vi "Vision Processing.vi"(8 "error in (no error)":errorcluster, 11 "Image Size":T2=enum."320x240") -> ()   [LabVIEW 2019]
uses:
  Vision Support Code/Camera Types.ctl
  <vilib>/Rock Robotics/WPI/Camera/WPI_CameraImageSize.ctl
  <vilib>/Rock Robotics/WPI/Camera/WPI_CameraWhite Balance Values.ctl
  <vilib>/Rock Robotics/WPI/Camera/WPI_CameraExposure Values.ctl
  <vilib>/Rock Robotics/WPI/Camera/WPI_CameraFrameRate.ctl
  Robot Global Data.vi
  <vilib>/Rock Robotics/Network Tables/NT Write Variant.vi
  <vilib>/vision/NI_Vision_Development_Module.lvlib
panel:
  out "Disqualified":i32
  out "Results":T1(array[cluster]) {"Normalized Center"."x" format="%#_2g"; "Normalized Center"."y" format="%#_2g"; "Overall Score" format="%#_2g"; "Distance (ft)" format="%#_3g"; "Area Score" format="%#_2g"; "Moment Score" format="%#_2g"; "Aspect Score" format="%#_2g"}
  in  "Size Limit %":dbl=0.04
  out "loop ms":u32
  in  "Display Original":bool
  in  "Display Mask":bool
  out "Instructions:":string="Connect a USB or IP camera to your roboRIO. If using a ring light and retroreflective tape, use Camera Settings outside the loop create a dark image with bright and colorful stripes. If used wihtout a ring light, brighten the images so that stripes are visible.\n\nLED Color can encoded as HSL or related color modes. Calibrate to the same color as the strips being reflected to the camera. Unlike the desktop example, this LED color must be set by hand. You can also put the calibration on the dashboard and send the LED Color to the RT code using Network Tables.\n\nThe Display buttons affects whether images are displayed on the panel. It takes quite a bit of CPU  to compress and transmit the images for display.\n\nAdjust Score Cutoff to make the code more or less picky. If the color is not very unique, you may need to increase the number of particles considered. The diagram uses a Size Limit to ignore colored things that are too small. You may need to adjust it if you are targetting from far away.\n\nResults give you the distance to the target, the center and box in a normalized (-1 to 1) and pixel coordinates.\n\nBe sure to read about setting camera exposure and brightness to help simplify your image and acquire color saturated images.\n\nThere are lots of comments on the diagram to explain the code."
  in  "Color Mode":u16(ring)=2 items=["RGB", "HSL", "HSV", "HSI"]
  in  "Particles":dbl=5.0
  in  "Score Cutoff %":dbl=75.0
  in  "Camera Type":T3=enum."MS HD3000 square"
  out "Qualified":i32
  in  "LED Color":T4={"Hue"={107.81818389892578, 139.81818389892578}, "Sat"={176.07142857142858, 255.0}, "Val"={40.53571428571429, 255.0}} {"Hue" scale=0.0..255.0 scale format="%#_3g"}
  out "Mask":T5(plugin-control)
  out "Original Image":T5(plugin-control)
  # "Scores"
  # "Good target, distance ft"
  # "Bad target"
  # "Score in %"
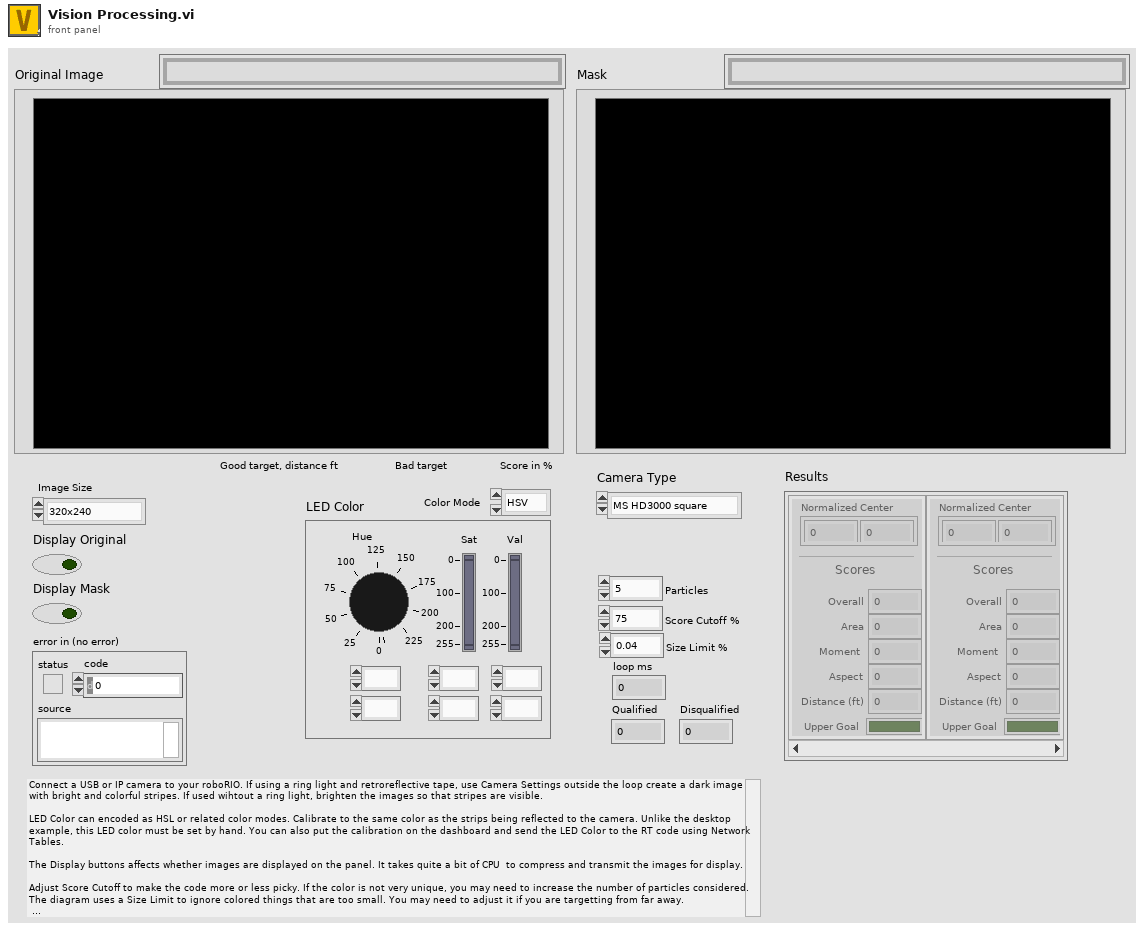
[diagram p1: front panel]
types:
  T1 = cluster{"diameter points":cluster{"first point":cluster{"x":dbl, "y":dbl}, "projected point":cluster{"x":dbl, "y":dbl}}, "Normalized Center":cluster{"x":dbl, "y":dbl}, "Overall Score":dbl, "Area Score":dbl, "Moment Score":dbl, "Aspect Score":dbl, "Distance (ft)":dbl, "Upper Goal":bool}[]
  T2 = typedef "WPI_CameraImageSize.ctl" = enum16{"640x480", "320x240", "160x120", "Custom"}
  T3 = typedef "Camera Types.ctl" = enum16{"206", "1011", "1013", "MS HD3000 square", "MS HD3000 640x480"}
  T4 = cluster{"Hue":cluster{dbl, dbl}, "Sat":cluster{dbl, dbl}, "Val":cluster{dbl, dbl}}
  T5 = typedef "IMAQ Image.ctl" = refnum<image>
  T6 = typedef "WPI_CameraFrameRate.ctl" = u32
  T7 = typedef "WPI_CameraExposure Values.ctl" = enum16{"Auto", "Flicker-free 50 Hz", "Flicker-free 60 Hz", "Hold current", "Custom"}
  T8 = typedef "WPI_CameraWhite Balance Values.ctl" = enum16{"Auto", "Fixed indoor", "Fixed outdoor 1", "Fixed outdoor 2", "Fixed fluorescent 1", "Fixed fluorescent 2", "Hold current", "Custom"}
  T9 = typedef "Particle Parameters" = i32
  T10 = typedef "Image Type" = u32
  T11 = typedef "WPI_CameraDevRef.ctl" = cluster{"Camera Address":string, "CameraStatus":errorcluster}
  T12 = cluster{"remainder":i32, "size":bool, "count":bool}
  T13 = typedef "Target Fields.ctl" = cluster{"diameter points":cluster{"first point":cluster{"x":dbl, "y":dbl}, "projected point":cluster{"x":dbl, "y":dbl}}, "normalized center":cluster{"x":dbl, "y":dbl}, "Overall Score":dbl, "Area Score":dbl, "Moment Score":dbl, "Aspect Score":dbl, "Distance (ft)":dbl, "Upper Goal":bool}
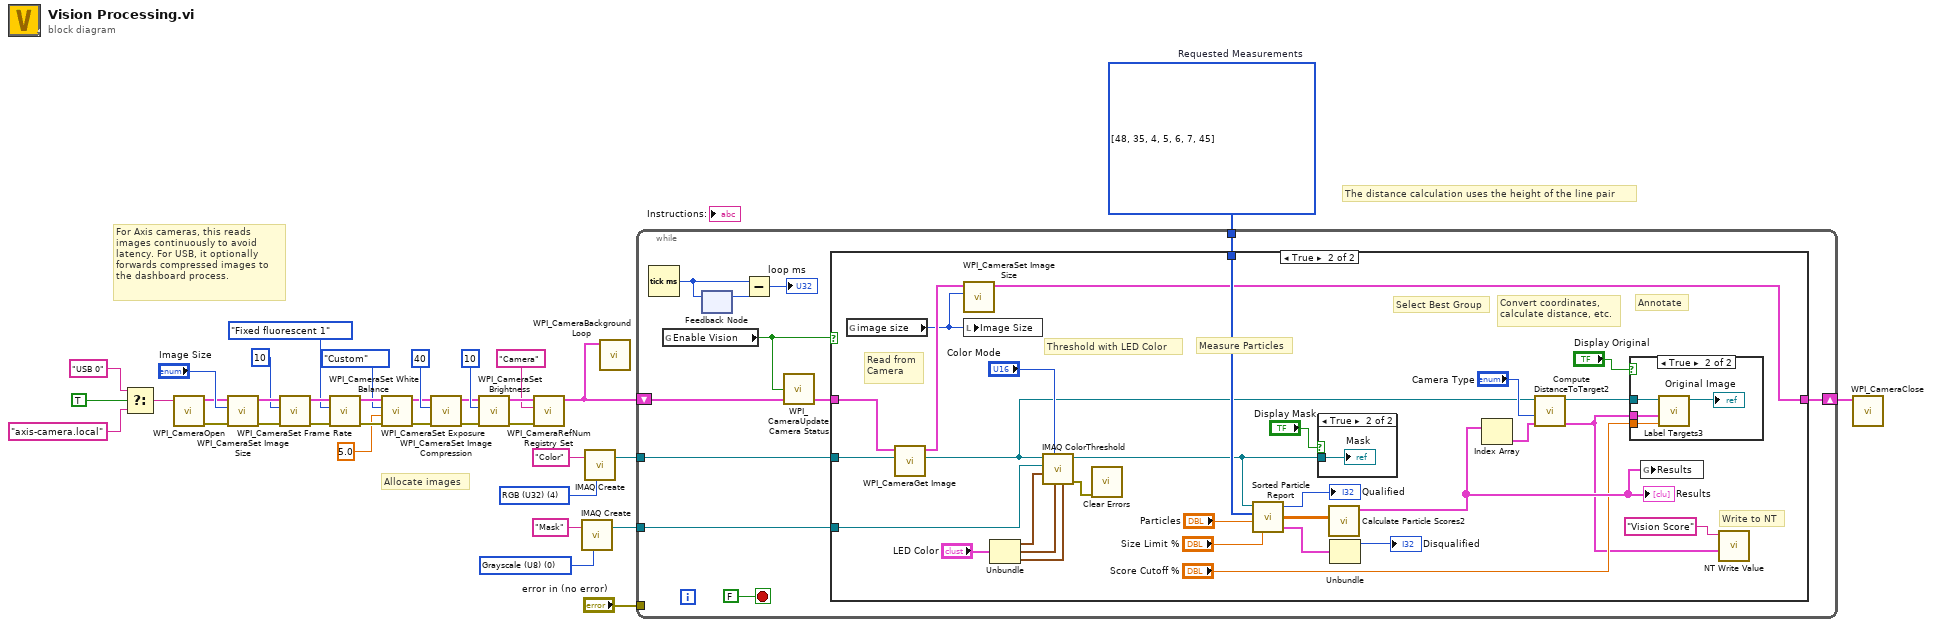
[diagram p0: block diagram]
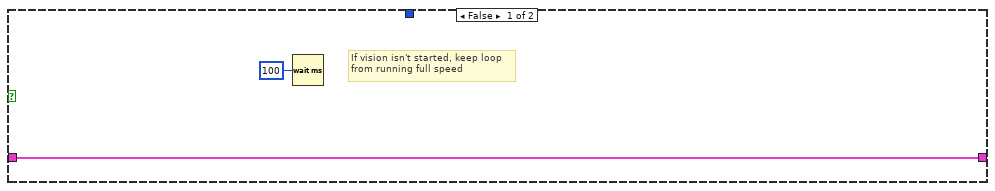
[diagram p2: hidden frame]
diagram:
  w31 = T9[] [48, 35, 4, 5, 6, 7, 45] items=["Center of Mass X", "Center of Mass Y", "First Pixel X", "First Pixel Y", "Bounding Rect Left", "Bounding Rect Top", "Bounding Rect Right", "Bounding Rect Bottom", "Max Feret Diameter Start X", "Max Feret Diameter Start Y", "Max Feret Diameter End X", "Max Feret Diameter End Y", "Max Horiz. Segment Length Left", "Max Horiz. Segment Length Right", "Max Horiz. Segment Length Row", "-", "Bounding Rect Width", "Bounding Rect Height", "Bounding Rect Diagonal", "Perimeter", "Convex Hull Perimeter", "Holes' Perimeter", "Max Feret Diameter", "Equivalent Ellipse Major Axis", "Equivalent Ellipse Minor Axis", "Equivalent Ellipse Minor Axis (Feret)", "Equivalent Rect Long Side", "Equivalent Rect Short Side", "Equivalent Rect Diagonal", "Equivalent Rect Short Side (Feret)", "Average Horiz. Segment Length", "Average Vert. Segment Length", "Hydraulic Radius", "Waddel Disk Diameter", "-", "Area", "Holes' Area", "Particle & Holes' Area", "Convex Hull Area", "Image Area", "-", "Number of Holes", "Number of Horiz. Segments", "Number of Vert. Segments", "-", "Orientation", "Max Feret Diameter Orientation", "-", "% Area/Image Area", "% Area/(Particle & Holes' Area)", "Ratio of Equivalent Ellipse Axes", "Ratio of Equivalent Rect Sides", "-", "Elongation Factor", "Compactness Factor", "Heywood Circularity Factor", "Type Factor", "-", "Sum X", "Sum Y", "Sum XX", "Sum XY", "Sum YY", "Sum XXX", "Sum XXY", "Sum XYY", "Sum YYY", "-", "Moment of Inertia XX", "Moment of Inertia XY", "Moment of Inertia YY", "Moment of Inertia XXX", "Moment of Inertia XXY", "Moment of Inertia XYY", "Moment of Inertia YYY", "Norm. Moment of Inertia XX", "Norm. Moment of Inertia XY", "Norm. Moment of Inertia YY", "Norm. Moment of Inertia XXX", "Norm. Moment of Inertia XXY", "Norm. Moment of Inertia XYY", "Norm. Moment of Inertia YYY", "Hu Moment 1", "Hu Moment 2", "Hu Moment 3", "Hu Moment 4", "Hu Moment 5", "Hu Moment 6", "Hu Moment 7"]  # Requested Measurements
  w34 = T10 0 items=["Grayscale (U8)", "Grayscale (I16)", "Grayscale (SGL)", "Complex (CSG)", "RGB (U32)", "HSL (U32)", "RGB (U64)", "Grayscale (U16)"] ("Image Type")
  w35 = T10 4 items=["Grayscale (U8)", "Grayscale (I16)", "Grayscale (SGL)", "Complex (CSG)", "RGB (U32)", "HSL (U32)", "RGB (U64)", "Grayscale (U16)"] ("Image Type")
  # "For Axis cameras, this reads\nimages continuously to avoid\nlatency. For USB, it optionally\nforwards compressed images to\nthe dashboard process."
  # "The distance calculation uses the height of the line pair"
  # "Allocate images"
  n1 = Select(t="USB 0" ("format string"), s=TRUE ("dot notation? (F)"), f="axis-camera.local" ("format string")) -> (s? t:f=w5:string)
  n2 = call <vilib>:"WPI_CameraOpen.vi"("Camera Address"=w5) -> ("error out"=w17:errorcluster, "CameraDevRef"=w18:T11)  [unwired: 1 in, 8 out]
  n3 = call <vilib>:"WPI_CameraSet Image Size.vi"("error in (no error)"=w17, "Image Size"="Image Size", "CameraDevRef"=w18) -> ("error out"=w16:errorcluster, "CameraDevRef Out"=w19:T11)  [unwired: 1 in, 6 out]
  n4 = call <vilib>:"WPI_CameraSet Frame Rate.vi"("error in (no error)"=w16, "Frame Rate (fps)"=T6 10, "CameraDevRef"=w19) -> ("error out"=w15:errorcluster, "CameraDevRef Out"=w21:T11)  [unwired: 7 out]
  n5 = call <vilib>:"WPI_CameraSet White Balance.vi"("error in (no error)"=w15, "White Balance"=WPI_CameraWhite_Balance_Values."Fixed fluorescent 1", "CameraDevRef"=w21) -> ("error out"=w14:errorcluster, "CameraDevRef Out"=w20:T11)  [unwired: 1 in, 6 out]
  n6 = call <vilib>:"WPI_CameraSet Exposure.vi"("error in (no error)"=w14, "Exposure (%)"=5.0, "Exposure"=WPI_CameraExposure_Values."Custom", "CameraDevRef"=w20) -> ("error out"=w13:errorcluster, "CameraDevRef Out"=w23:T11)  [unwired: 6 out]
  n7 = call <vilib>:"WPI_CameraSet Image Compression.vi"("error in (no error)"=w13, "Compression"=40, "CameraDevRef"=w23) -> ("error out"=w12:errorcluster, "CameraDevRef Out"=w22:T11)  [unwired: 7 out]
  n8 = call <vilib>:"WPI_CameraSet Brightness.vi"("error in (no error)"=w12, "Brightness"=10, "CameraDevRef"=w22) -> ("error out"=w11:errorcluster, "CameraDevRef Out"=w29:T11)  [unwired: 1 in, 6 out]
  n9 = call <vilib>:"WPI_CameraRefNum Registry Set.vi"("error in (no error)"=w11, "refnum name"="Camera", "CameraDevRef"=w29) -> ("CameraDevRef"=w4:T11)  [unwired: 1 in, 7 out]
  n10 = call "IMAQ Create"("Image Name"="Mask", "Image Type"=w34) -> ("New Image"=w32:T5)  [unwired: 2 in, 2 out]
  n11 = call "IMAQ Create"("Image Name"="Color", "Image Type"=w35) -> ("New Image"=w30:T5)  [unwired: 2 in, 2 out]
  n12 = call <vilib>:"WPI_CameraBackground Loop.vi"("CameraDevRef"=w4) -> ()  [unwired: 11 in]
  n13 = while {
    tunnel: w30 -> [w44]
    tunnel: w32 -> [w46]
    tunnel: w31 -> [w45]
    shift-right: [w43] -> w3
    shift-left: w4 -> [w42]
    tunnel: "error in (no error)" -> [_]
    stop <- FALSE stop-if-true
    n14 = Tick Count (ms)() -> (millisecond timer value=w38:u32)
    n15 = global read "Robot Global Data.vi" "Enable Vision"() -> (w40:bool)
    n16 = feedback #1() -> (w39:u32)  [unwired: 1 in]
    n17 = feedback-in #1(w38) -> ()
    n18 = Subtract(x=w38, y=w39) -> (x-y=→"loop ms":u32)
    n19 = call <vilib>:"WPI_CameraUpdate Camera Status.vi"("CameraDevRef In"=w42, "Enable Vision"=w40) -> ("CameraDevRef Out"=w41:T11)  [unwired: 3 in]
    n20 = case shown="True" w40 {
      tunnel: w46 -> [_ w79]
      tunnel: w45 -> [_ w75]
      tunnel: w41 -> [w49 w67]
      tunnel: w44 -> [_ w66]
      tunnel: [w49 w61] -> w43
      frame False {
        # "If vision isn't started, keep loop\nfrom running full speed"
        n21 = Wait (ms)(milliseconds to wait=u32 100) -> ()  [unwired: 1 out]
      }
      frame True {
        # "Write to NT"
        # "Read from\nCamera"
        # "Measure Particles"
        # "Convert coordinates,\ncalculate distance, etc."
        # "Annotate"
        # "Select Best Group"
        # "Threshold with LED Color"
        n22 = global read "Robot Global Data.vi" "image size"() -> (w60:T2)
        n23 = call <vilib>:"WPI_CameraGet Image.vi"("Image"=w66, "CameraDevRef"=w67) -> ("Image Out"=w65:T5, "CameraDevRef Out"=w62:T11)  [unwired: 7 in, 1 out]
        n24 = call <vilib>:"WPI_CameraSet Image Size.vi"("Image Size"=w60, "CameraDevRef"=w62) -> ("CameraDevRef Out"=w61:T11)  [unwired: 2 in, 7 out]
        n25 = local write "Image Size"(w60) -> ()
        n26 = Unbundle("LED Color") -> ("Hue"=w78:cluster{dbl, dbl}, "Sat"=w77:cluster{dbl, dbl}, "Val"=w76:cluster{dbl, dbl})
        n27 = call "IMAQ ColorThreshold"("Blue or Luma or Val or Inten Range"=w76, "Green or Sat Range"=w77, "Color Mode"="Color Mode", "Red or Hue Range"=w78, "Image Dst"=w79, "Image Src"=w65) -> ("error out"=w73:errorcluster, "Image Dst Out"=w71:T5)  [unwired: 4 in]
        n28 = call <vilib>:"Clear Errors.vi"("error in (no error)"=w73) -> ()  [unwired: 5 in, 2 out]
        n29 = call "Sorted Particle Report.vi"("Min Area Size %"="Size Limit %", "Particle Count Limit"="Particles", "Pixel Measurements"=w75, "Image in"=w71) -> ("limits"=w52:T12, "Sorted Data"=w58:dbl[][], "Particles"=→"Qualified":i32)
        n30 = case shown="True" "Display Mask" {
          tunnel: w71 -> [_ w80]
          frame False {
          }
          frame True {
            "Mask" <- w80
          }
        }
        n31 = call "Calculate Particle Scores2.vi"("Sorted Data"=w58) -> ("Scores"=w55:T13[])  [unwired: 10 in]
        "Results" <- w55
        n32 = Unbundle(w52) -> ("remainder"=→"Disqualified":i32)  [unwired: 2 out]
        n33 = Index Array(array=w55) -> (element=w56:T13)  [unwired: 1 in]
        n34 = call "Compute DistanceToTarget2.vi"("results"=w56, "Camera Type"="Camera Type", "Image Src"=w65) -> ("results out"=w50:T13, "Image Dst Out"=w57:T5)  [unwired: 7 in]
        n35 = case shown="True" "Display Original" {
          tunnel: w57 -> [_ w83]
          tunnel: w50 -> [_ w82]
          tunnel: "Score Cutoff %" -> [_ w81]
          frame False {
          }
          frame True {
            n36 = call "Label Targets3.vi"("Score Threshold"=w81, "results"=w82, "Image in"=w83) -> ("Image out"=→"Original Image":T5)  [unwired: 8 in]
          }
        }
        n37 = global write "Robot Global Data.vi" "Results"(w55) -> ()
        n38 = call-poly <vilib>:"NT Write Value.vi"("Variant"=w50, "Name"="Vision Score") -> ()  [unwired: 9 in, 1 out]
      }
    }
  }
  n39 = call <vilib>:"WPI_CameraClose.vi"("CameraDevRef"=w3) -> ()  [unwired: 1 in, 10 out]
